vi "IsFirst.vi"(8 "error in (no error)":errorcluster, 10 "BC ID":i32, 11 "BCReg":refnum<data-value>) -> (0 "error out":errorcluster, 1 "First?":bool, 2 "Found?":bool, 3 "BCReg":refnum<data-value>)   [LabVIEW 2014, in "BusController.lvlib" / "BCReg.lvclass"]
uses:
  BCReg.lvclass
  BCReg.lvclass/BCReg.ctl
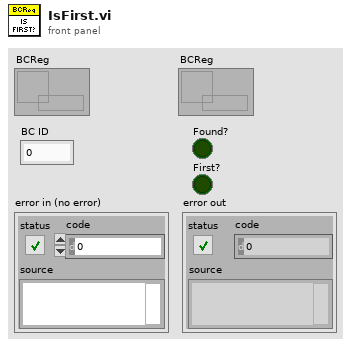
[diagram p1: front panel]
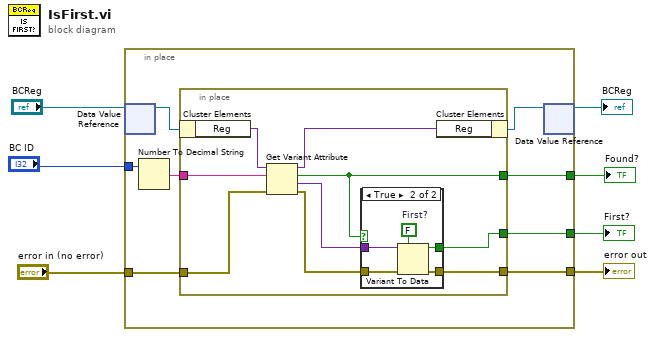
[diagram p0: block diagram]
diagram:
  n1 = in-place {
    in-place-border: "BC ID" -> [w15]
    in-place-border: [w13] -> w3
    in-place-border: [w12] -> w2
    in-place-border: [w11] -> w1
    in-place-border: "error in (no error)" -> [w10]
    n2 = in-place-dvr #1("BCReg") -> (w9:refnum<class "BCReg.lvclass">)  [unwired: 1 out]
    n3 = Number To Decimal String(number=w15) -> (decimal integer string=w14:string)  [unwired: 1 in]
    n4 = in-place {
      in-place-border: w14 -> [w24]
      in-place-border: [w22] -> w13
      in-place-border: [w19] -> w12
      in-place-border: [w18] -> w11
      in-place-border: w10 -> [w17]
      n5 = in-place-cluster #2(w9) -> ("Reg"=w23:variant)
      n6 = Get Variant Attribute(Variant=w23, name=w24, error in=w17) -> (duplicate Variant=w16:variant, found=w22:bool, value=w21:variant, error out=w20:errorcluster)  [unwired: 1 in]
      n7 = case shown="True" w22 {
        tunnel: w21 -> [_ w30]
        tunnel: w20 -> [w25 w29]
        tunnel: [_ w27] -> w19
        tunnel: [w25 w26] -> w18
        frame False {
        }
        frame True {
          w28 = FALSE  # First?
          n8 = Variant To Data(error in=w29, type=w28, Variant=w30) -> (data=w27:bool, error out=w26:errorcluster)
        }
      }
      n9 = in-place-cluster #2("Reg"=w16) -> (w8:refnum<class "BCReg.lvclass">)
    }
    n10 = in-place-dvr #1(w8) -> (→"BCReg":refnum<data-value>)  [unwired: 1 out]
  }
  "First?" <- w2
  "Found?" <- w3
  "error out" <- w1
